vi "Open SystemLink Connection (API Key).vi"(5 "SystemLink server base URL":string="https://", 7 "API Key":string, 11 "error in (no error)":errorcluster) -> (4 "SystemLink repo out":T1, 15 "error out":errorcluster)   [LabVIEW 2025, in "SystemLink_Repo_API.lvlib"]
doc: "Opens an HTTP client handle and passes on the SystemLink server base URL.\n\nInputs:\nSystemLink server base URL- Specifies the base URL of the SystemLink server to connect with (e.g. https://192.168.10.15, https://mysystemlinkserver.com)\nUsername - Specify the SystemLink username\nPassword - Specify the SystemLink password\n\nOutput:\nSystemLink repo out - pass this wire to all the other VIs in this SystemLink Repo API."
uses:
  SystemLink_Repo_API.lvlib
  _support/systemlink repo.ctl
  <vilib>/httpClient/ClientHandle.ctl
  <vilib>/httpClient/LabVIEWHTTPClient.lvlib
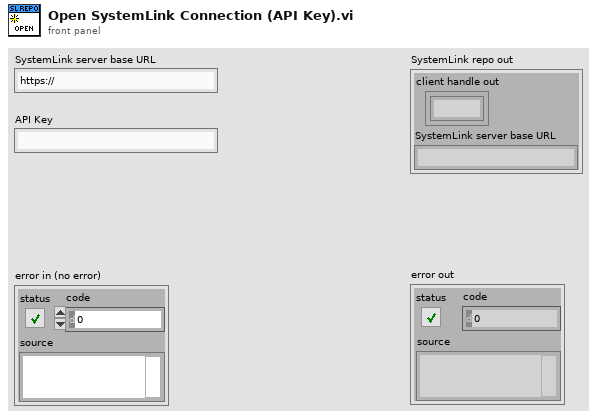
[diagram p1: front panel]
types:
  T1 = typedef "SystemLink_Repo_API.lvlib/systemlink repo.ctl" = cluster{"client handle out":T2, "SystemLink server base URL":string}
  T2 = typedef "LabVIEWHTTPClient.lvlib/ClientHandle.ctl" = refnum<k1>
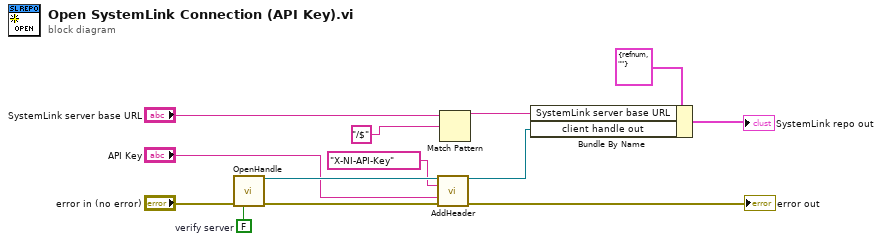
[diagram p0: block diagram]
diagram:
  w9 = FALSE  # verify server
  n1 = call <vilib>:"OpenHandle.vi"("error in (no error)"="error in (no error)", "verify server(true)"=w9) -> ("client handle out"=w4:T2, "error out"=w10:errorcluster)  [unwired: 12 in]
  n2 = call <vilib>:"AddHeader.vi"("client handle"=w4, "header"="X-NI-API-Key", "value"="API Key", "error in (no error)"=w10) -> ("client handle out"=w3:T2, "error out"=→"error out":errorcluster)  [unwired: 10 in]
  n3 = Match Pattern(string="SystemLink server base URL", regular expression="/$") -> (before substring=w7:string)  [unwired: 1 in, 3 out]
  n4 = Bundle By Name(cluster=T1 {"client handle out"=refnum, "SystemLink server base URL"=""} ("SystemLink repo out"), "SystemLink server base URL"=w7, "client handle out"=w3) -> (→"SystemLink repo out":T1)
